vi "Continuous Acquisition.vi"() -> ()   [LabVIEW 2020]
uses:
  <vilib>/DAQmx/read.llb/DAQmx Read (Analog 2D DBL NChan NSamp).vi
  <vilib>/DAQmx/create/channels.llb/DAQmx Create Channel (AI-Voltage-Basic).vi
  <vilib>/DAQmx/configure/timing.llb/DAQmx Timing (Sample Clock).vi
  <vilib>/DAQmx/miscellaneous.llb/DAQmx Fill In Error Info.vi
  <resource>/objmgr/daqmx.rc
panel:
  out "Waveform Chart":dbl[][](graph)
  in  "stop":bool
  out "Samples in Buffer":i32
  out "Boolean":bool
  in  "Buffer Read Rate":u32
  in  "Buffer size (sample per channel)":i32=1000
  in  "rate":dbl=1000.0 format="%0.2f"
  in  "DAQmx Physical Channel":tag
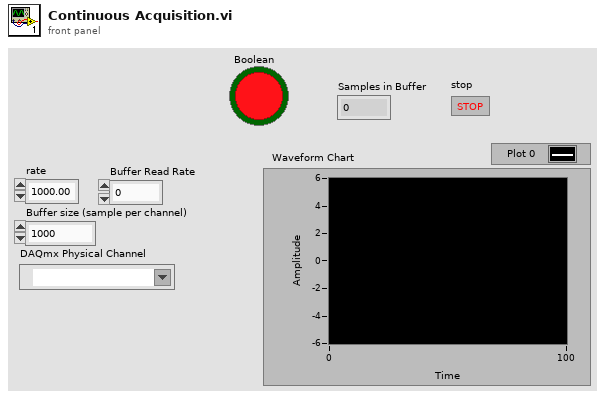
[diagram p1: front panel]
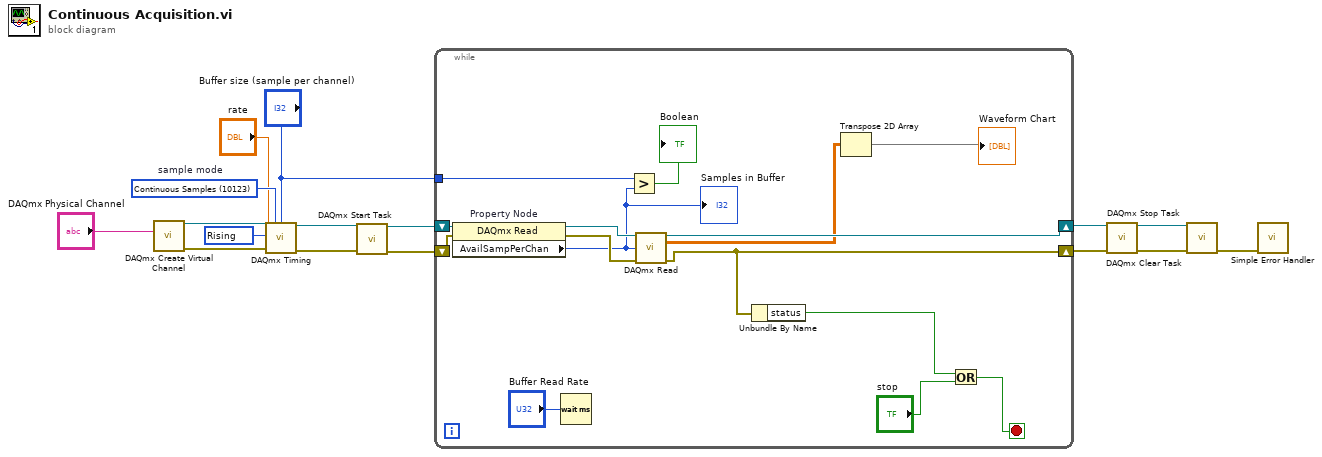
[diagram p0: block diagram]
diagram:
  w2 = 10280 items=["Rising"=10280, "Falling"=10171] ("active edge")
  w13 = 10123 items=["Finite Samples"=10178, "Continuous Samples"=10123, "Hardware Timed Single Point"=12522]  # sample mode
  n1 = call-poly <vilib>:"DAQmx Create Virtual Channel.vi"("physical channels"="DAQmx Physical Channel") -> ("task out"=w15:refnum<k21>, "error out"=w14:errorcluster)  [unwired: 13 in]
  n2 = call-poly <vilib>:"DAQmx Timing.vi"("task/channels in"=w15, "sample mode"=w13, "samples per channel"="Buffer size (sample per channel)", "rate"="rate", "active edge"=w2, "error in"=w14) -> ("task out"=w11:refnum<k21>, "error out"=w10:errorcluster)  [unwired: 8 in]
  n3 = call <vilib>:"DAQmx Start Task.vi"("task/channels in"=w11, "error in"=w10) -> ("task out"=w9:refnum<k21>, "error out"=w8:errorcluster)  [unwired: 12 in]
  n4 = while {
    tunnel: "Buffer size (sample per channel)" -> [w26]
    shift-right: [w19] -> w6
    shift-left: w9 -> [w31]
    shift-right: [w20] -> w5
    shift-left: w8 -> [w30]
    stop <- w22 stop-if-true
    n5 = property on="Property Node" class="DAQmx Read"(reference=w31, error in=w30) -> (reference out=w29:refnum<k21>, error out=w28:errorcluster, "AvailSampPerChan"=w24:u32)
    "Samples in Buffer" <- w24
    n6 = Wait (ms)(milliseconds to wait="Buffer Read Rate") -> ()  [unwired: 1 out]
    n7 = Greater?(x=w26, y=w24) -> (0:→"Boolean":bool)
    n8 = call-poly <vilib>:"DAQmx Read.vi"("task/channels in"=w29, "number of samples per channel"=w24, "error in"=w28) -> ("task out"=w19:refnum<k21>, "data"=w18:dbl[][], "error out"=w20:errorcluster)  [unwired: 10 in]
    n9 = Unbundle By Name(w20) -> ("status"=w23:bool)
    n10 = Transpose 2D Array(2D array=w18) -> (transposed array=→"Waveform Chart":dbl[][])
    n11 = Or(x=w23, y="stop") -> (x .or. y?=w22:bool)
  }
  n12 = call <vilib>:"DAQmx Stop Task.vi"("task/channels in"=w6, "error in"=w5) -> ("task out"=w4:refnum<k21>, "error out"=w3:errorcluster)  [unwired: 12 in]
  n13 = call <vilib>:"DAQmx Clear Task.vi"("task in"=w4, "error in"=w3) -> ("error out"=w1:errorcluster)  [unwired: 13 in]
  n14 = call <vilib>:"Simple Error Handler.vi"("error in (no error)"=w1) -> ()  [unwired: 4 in, 5 out]
